vi "普通cable读写操作_old.vi"(8 "input_data":u8[](array[numeric]) format="%.0x", 9 "input_mode":string(combo), 10 "Channel":u8 max=5 step=1, 11 "VISA":refnum<visa-resource-name>="COM6") -> (2 "result":bool, 3 "data read":u8[](array[numeric]) format="%.0x")   [LabVIEW 2011]
panel:
  out "message":string
  in  "address":u8
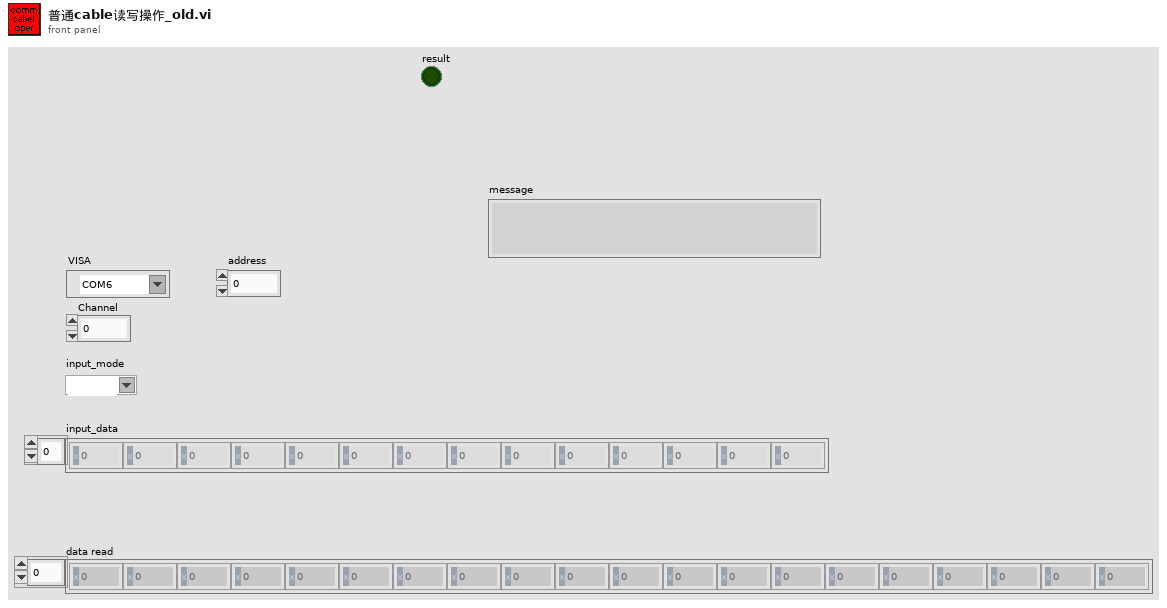
[diagram p1: front panel]
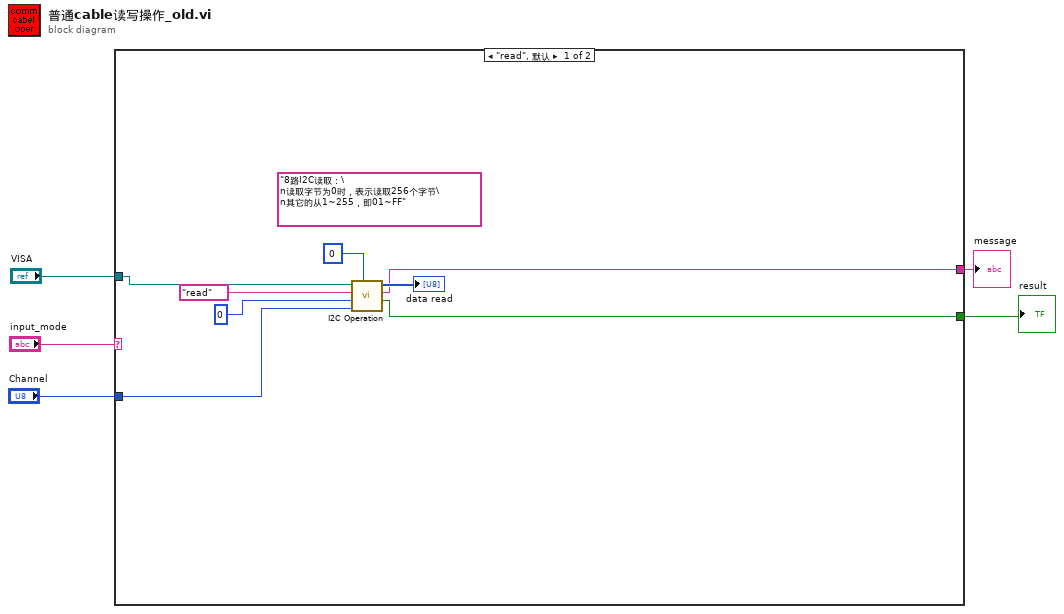
[diagram p0: block diagram]
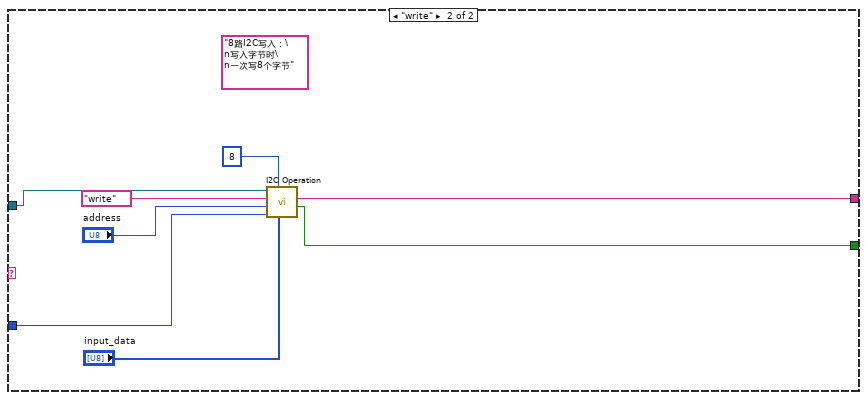
[diagram p2: hidden frame]
diagram:
  n1 = case shown="\"read\", 默认" "input_mode" {
    tunnel: "VISA" -> [w13 w21]
    tunnel: "Channel" -> [w9 w17]
    tunnel: [w7 w15] -> w2
    tunnel: [w6 w14] -> w1
    frame "read", Default {
      (unwired) "8路I2C读取：\n读取字节为0时，表示读取256个字节\n其它的从1~255，即01~FF"
      n2 = call "I2C Operation.vi"("size"=0, "Channel"=w9, "address"=u8 0, "mode"="read", "VISA"=w13) -> ("result"=w6:bool, "message"=w7:string, "Data Out"=→"data read":u8[])  [unwired: 4 in]
    }
    frame "write" {
      (unwired) "8路I2C写入：\n写入字节时\n一次写8个字节"
      n3 = call "I2C Operation.vi"("input_data"="input_data", "size"=8, "Channel"=w17, "address"="address", "mode"="write", "VISA"=w21) -> ("result"=w14:bool, "message"=w15:string)  [unwired: 3 in, 1 out]
    }
  }
  "message" <- w2
  "result" <- w1
